vi "Close Log.vi"(8 "error in (no error)":errorcluster, 11 "LogRotate in":refnum<class "LogRotate.lvclass">) -> (0 "error out":errorcluster, 3 "LogRotate out":refnum<class "LogRotate.lvclass">)   [LabVIEW 2021, in "Error_Manager.lvlib" / "LogRotate.lvclass"]
uses:
  LogRotate.lvclass
  LogRotate.lvclass/LogRotate.ctl
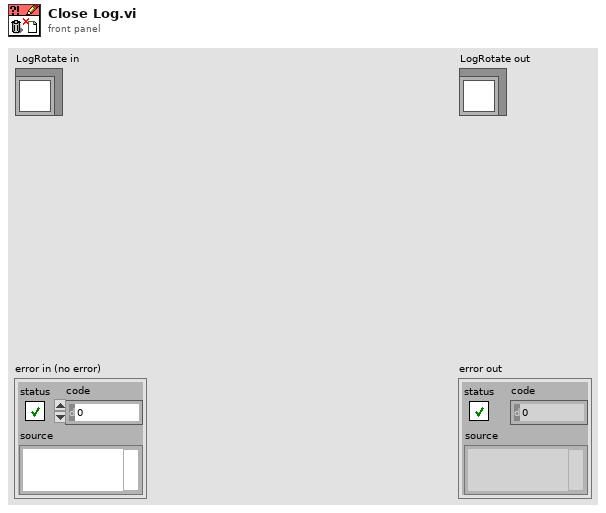
[diagram p1: front panel]
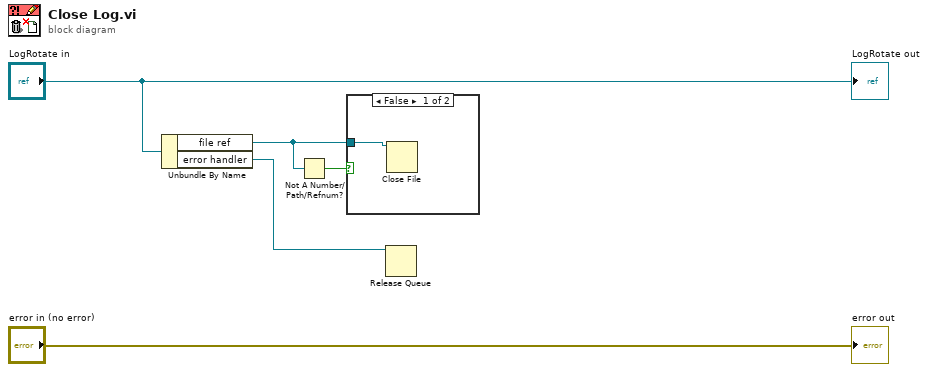
[diagram p0: block diagram]
diagram:
  n1 = Unbundle By Name("LogRotate in") -> ("file ref"=w3:refnum<file>, "error handler"=w1:refnum<queue>)
  n2 = Not A Number/Path/Refnum?(number/path/refnum=w3) -> (NaN/Path/Refnum?=w2:bool)
  n3 = case shown="False" w2 {
    tunnel: w3 -> [w6 _]
    frame False {
      n4 = Close File(refnum=w6) -> ()  [unwired: 1 in, 2 out]
    }
    frame True {
    }
  }
  n5 = Release Queue(queue=w1) -> ()  [unwired: 2 in, 3 out]
  "error out" <- "error in (no error)"
  "LogRotate out" <- "LogRotate in"
